vi "StrBin_To_ArrayBool_8Bit.vi"(11 "StrBin":string="0000000000") -> (1 "Err":bool, 3 "Out":bool[](array[boolean]))   [LabVIEW 2018]
panel:
  out "length":i32
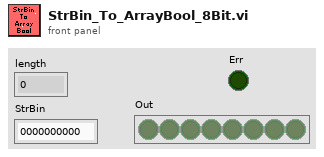
[diagram p1: front panel]
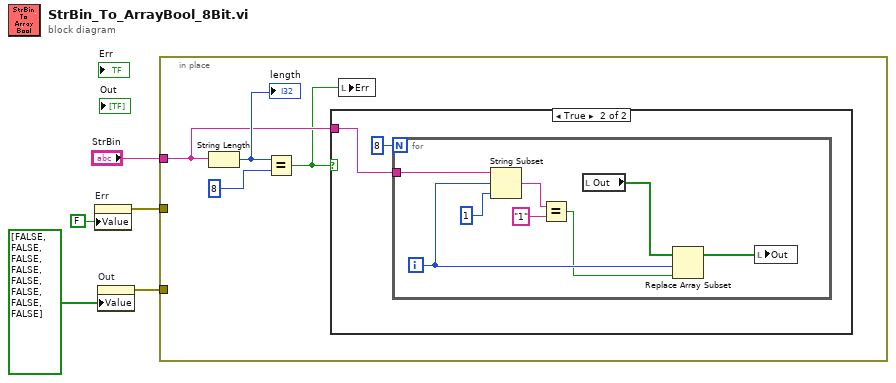
[diagram p0: block diagram]
diagram:
  n1 = property on="Err" class="Bool (strict)"("Value"=FALSE ("Err")) -> (error out=w2:errorcluster)  [unwired: 2 in, 1 out]
  n2 = property on="Out" class="Arr (strict)"("Value"=bool[] [FALSE, FALSE, FALSE, FALSE, FALSE, FALSE, FALSE, FALSE] ("Out")) -> (error out=w4:errorcluster)  [unwired: 2 in, 1 out]
  n3 = in-place {
    in-place-border: "StrBin" -> [w7]
    in-place-border: w4 -> [_]
    in-place-border: w2 -> [_]
    n4 = String Length(string=w7) -> (length=w9:i32)
    "length" <- w9
    n5 = Equal?(x=w9, y=8) -> (x = y?=w6:bool)
    n6 = case shown="True" w6 {
      tunnel: w7 -> [_ w11]
      frame False {
      }
      frame True {
        n7 = for {
          N: 8 -> [_]
          tunnel: w11 -> [w19]
          i -> [w13]
          n8 = String Subset(string=w19, offset (0)=w13, length (rest)=1 ("length (rest)")) -> (substring=w17:string)
          n9 = Equal?(x=w17, y="1") -> (x = y?=w12:bool)
          n10 = local read "Out"() -> (w15:bool[])
          n11 = Replace Array Subset(array=w15, new element=w12, index=w13) -> (w14:bool[])
          n12 = local write "Out"(w14) -> ()
        }
      }
    }
    n13 = local write "Err"(w6) -> ()
  }
